vi "uActor_Core.vi"(8 "error in (no error)":errorcluster, 11 "Test_uActor_Echo in":refnum<class "Test_uActor_Echo.lvclass">) -> (0 "error out":errorcluster, 3 "Test_uActor_Echo out":refnum<class "Test_uActor_Echo.lvclass">)   [LabVIEW 2021, in "Test_uActor_Echo.lvclass"]
doc: "Dynamic dispatch method to allow children to add helper loops when desired."
uses:
  Test_uActor_Echo.lvclass
  Test_uActor_Echo.lvclass/Test_uActor_Echo.ctl
  Bin/uFramework.lvlibp/uActor/uActor.lvclass
panel:
  out "Received":string
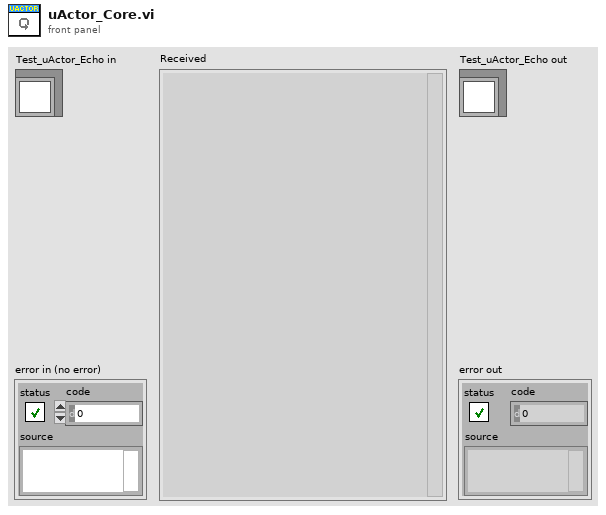
[diagram p1: front panel]
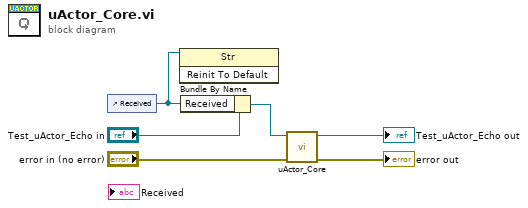
[diagram p0: block diagram]
diagram:
  n1 = control-ref of="Received"() -> (w1:refnum<vi>)
  n2 = invoke class="Str" method="Reinit To Default"(reference=w1) -> ()  [unwired: 2 in, 3 out]
  n3 = Bundle By Name(cluster="Test_uActor_Echo in", "Received"=w1) -> (w2:refnum<class "Test_uActor_Echo.lvclass">)
  n4 = call-parent "uActor_Core.vi"("error in (no error)"="error in (no error)", "uActor in"=w2) -> ("error out"=→"error out":errorcluster, "uActor out"=→"Test_uActor_Echo out":refnum<class "Test_uActor_Echo.lvclass">)  [unwired: 8 in]
